vi "getHumidity.vi"(8 "error in (no error)":errorcluster, 11 "WeatherData in":refnum<class "WeatherData.lvclass">) -> (0 "error out":errorcluster, 2 "Humidity":dbl, 3 "WeatherData out":refnum<class "WeatherData.lvclass">)   [LabVIEW 2016, in "WeatherData.lvclass"]
uses:
  WeatherData.lvclass
  WeatherData.lvclass/WeatherData.ctl
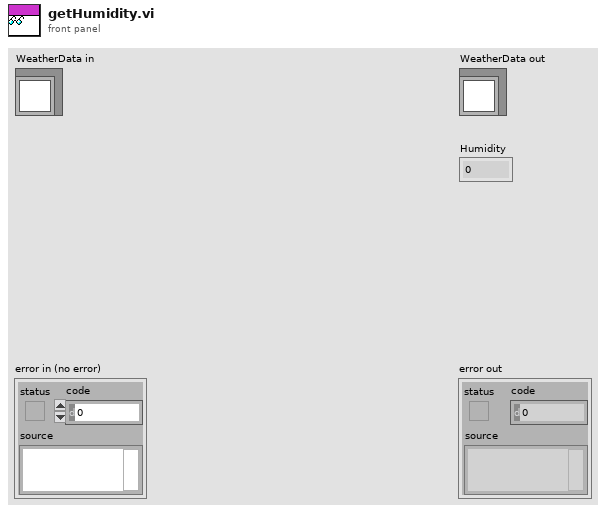
[diagram p1: front panel]
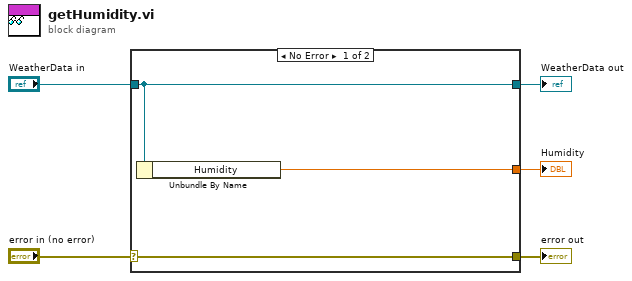
[diagram p0: block diagram]
diagram:
  n1 = case shown="No Error" "error in (no error)" {
    selector: "error in (no error)" -> [w8 w9]
    tunnel: [w8 w9] -> w4
    tunnel: [w7 w10] -> w2
    tunnel: "WeatherData in" -> [w7 w10]
    tunnel: [w6 _] -> w1
    frame No Error {
      n2 = Unbundle By Name(w7) -> ("Humidity"=w6:dbl)
    }
    frame Error {
    }
  }
  "error out" <- w4
  "WeatherData out" <- w2
  "Humidity" <- w1
